vi "sendOutputData.vi"(8 "error in (no error)":errorcluster, 11 "Model in":refnum<class "Model.lvclass">) -> (0 "error out":errorcluster, 3 "Model out":refnum<class "Model.lvclass">)   [LabVIEW 2012, in "Model.lvclass"]
uses:
  Model.lvclass
  Model.lvclass/Model.ctl
  Program Files (x86)/National Instruments/LabVIEW 2012/user.lib/Common/SerialProtocols/SerialCommunicator/SerialCommunicator.lvclass
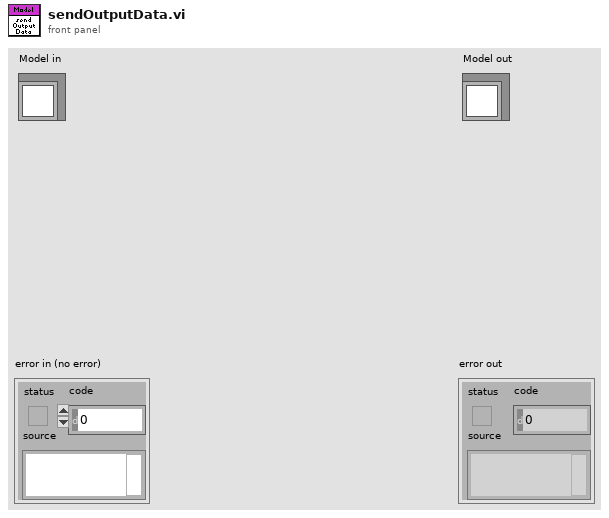
[diagram p1: front panel]
types:
  T1 = typedef "OutputData.ctl" = cluster{"Step & Direction":i16, "Blower RPM":u8, "PWM (SSR)":u8, "Ch1":u16, "Ch2":u16, "Ch3":u16, "Ch4":u16}
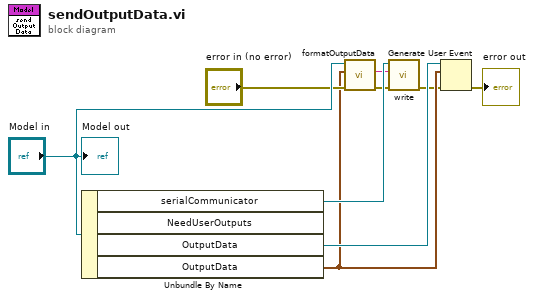
[diagram p0: block diagram]
diagram:
  n1 = Unbundle By Name("Model in") -> ("serialCommunicator"=w8:refnum<class "SerialCommunicator.lvclass">, "OutputData"=w4:refnum<user-event>, "OutputData"=w3:T1)  [unwired: 1 out]
  n2 = call "formatOutputData.vi"("error in (no error)"="error in (no error)", "outputData"=w3, "Model in"="Model in") -> ("error out"=w5:errorcluster, "outputDataString"=w7:string)  [unwired: 6 in, 1 out]
  n3 = call-dynamic "write.vi"("error in (no error)"=w5, "writeString"=w7, "SerialCommunicator in"=w8) -> ("error out"=w2:errorcluster)  [unwired: 7 in, 1 out]
  n4 = Generate User Event(user event=w4, event data cluster=w3, error in=w2) -> (error out=→"error out":errorcluster)  [unwired: 1 out]
  "Model out" <- "Model in"
